vi "getEdgeLength.vi"(11 "StationKeeping in":refnum<class "StationKeeping.lvclass">) -> (1 "Edge Length":dbl, 3 "StationKeeping out":refnum<class "StationKeeping.lvclass">)   [LabVIEW 2011, in "StationKeeping.lvclass"]
doc: "Returns the length of one edge of the station (helpful for giving the scale of the station, to know, for example, how big a pattern to use for sailing inside the station)."
uses:
  StationKeeping.lvclass
  StationKeeping.lvclass/StationKeeping.ctl
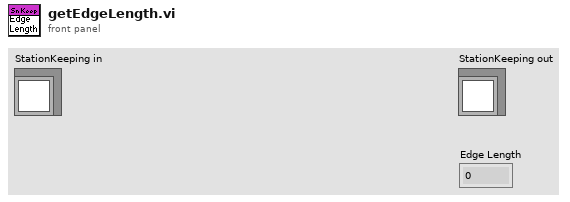
[diagram p1: front panel]
types:
  T1 = typedef "UTM Location.ctl" = cluster{"UTM Zone":dbl, "Hemisphere":enum16{"North", "South"}, "East":dbl, "North":dbl}
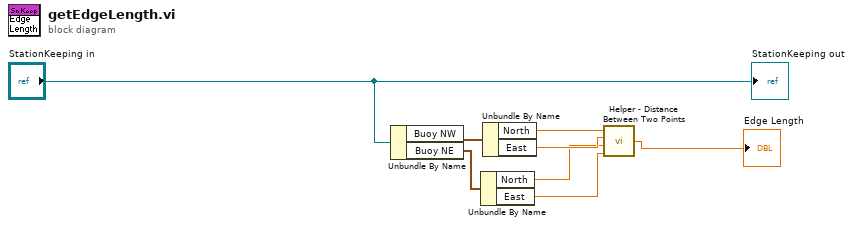
[diagram p0: block diagram]
diagram:
  n1 = Unbundle By Name("StationKeeping in") -> ("Buoy NW"=w6:T1, "Buoy NE"=w5:T1)
  n2 = Unbundle By Name(w5) -> ("North"=w2:dbl, "East"=w1:dbl)
  n3 = Unbundle By Name(w6) -> ("North"=w4:dbl, "East"=w3:dbl)
  n4 = call "Helper - Distance Between Two Points.vi"("y 2"=w1, "x 2"=w2, "y"=w3, "x"=w4) -> ("Numeric"=→"Edge Length":dbl)
  "StationKeeping out" <- "StationKeeping in"
